vi "Parse Xeryon STAT.vi"(11 "STAT Word":i32) -> (2 "STAT True":string, 3 "STAT":string[][](table))   [LabVIEW 2019, in "Inst UI.Xeryon-Rotator.lvclass"]
uses:
  Inst UI.Xeryon-Rotator.lvclass
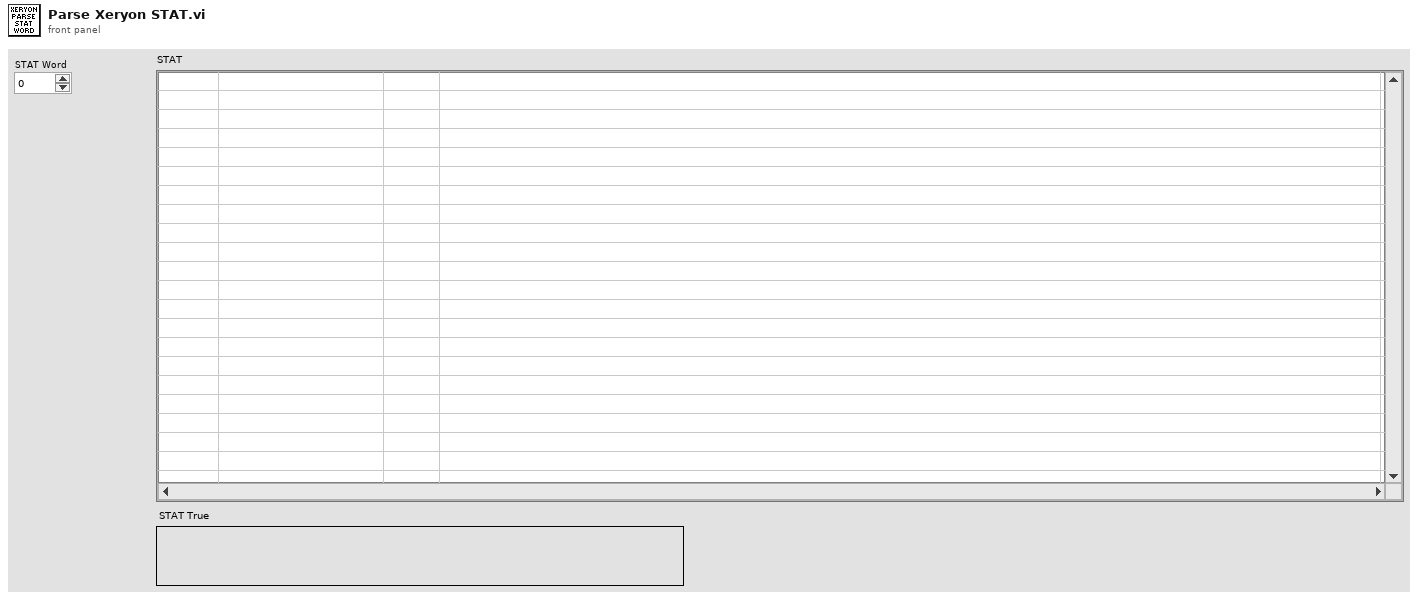
[diagram p1: front panel]
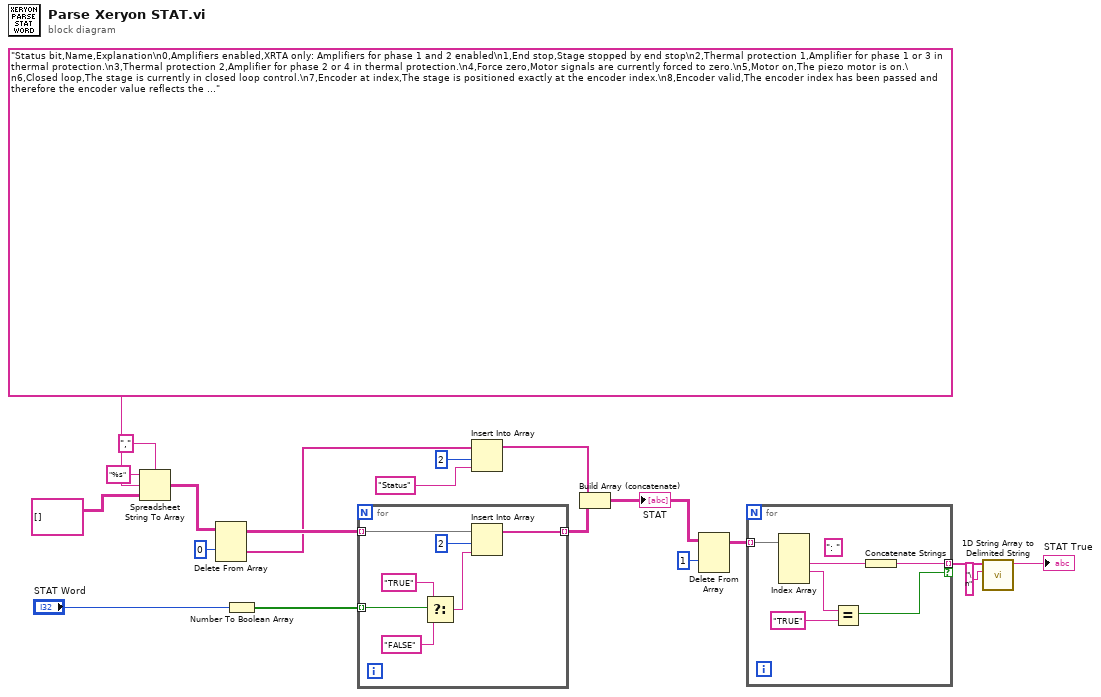
[diagram p0: block diagram]
diagram:
  n1 = Spreadsheet String To Array(delimiter (Tab)=",", format string="%s", spreadsheet string="Status bit,Name,Explanation\n0,Amplifiers enabled,XRTA only: Amplifiers for phase 1 and 2 enabled\n1,End stop,Stage stopped by end stop\n2,Thermal protection 1,Amplifier for phase 1 or 3 in thermal protection.\n3,Thermal protection 2,Amplifier for phase 2 or 4 in thermal protection.\n4,Force zero,Motor signals are currently forced to zero.\n5,Motor on,The piezo motor is on.\n6,Closed loop,The stage is currently in closed loop control.\n7,Encoder at index,The stage is positioned exactly at the encoder index.\n8,Encoder valid,The encoder index has been passed and therefore the encoder value reflects the absolute position and not the relative position with respect to the startup position.\n9,Searching index,The stage is currently searching the index position.\n10,Position reached,The target position is reached (within tolerance limits).\n11,Error compensation,Error compensation is on.\n12,Encoder error,There is an error produced by the encoder.\n13,Scanning,The stage is in a scanning mode.\n14,Left end stop,The left end stop is passed.\n15,Right end stop,The right end stop is passed.\n16,Error limit,The position error has reached the limit set by ELIM. This can indicate a collision or mechanical limit (end of stroke).\n17,Searching optimal frequency,The driver is searching for the optimal excitation frequency of the piezo motor.\n18,Safety timeout triggered,The safety timeout was triggered. See the explanation of the command 'TOU2'.\n19,EtherCAT acknowledge,Used when control via EtherCAT\n20,Emergency stop,not used\n21,Position fail,The safety timeout TOU3 was triggered.", array type (2D Dbl)=string[][] [] ("2-D Array")) -> (array=w5:string[][])
  n2 = Delete From Array(array=w5, index (row)=0) -> (deleted portion=w18:string[], array with subset deleted=w19:string[][])  [unwired: 2 in]
  n3 = Number To Boolean Array(number="STAT Word") -> (Boolean array=w2:bool[])
  n4 = for {
    tunnel: w19 -> [w24] mode=indexing
    tunnel: w2 -> [w27] mode=indexing
    tunnel: [w21] -> w14 mode=indexing
    n5 = Select(t="TRUE", s=w27, f="FALSE") -> (s? t:f=w23:string)
    n6 = Insert Into Array(array=w24, index=2, new element=w23) -> (w21:string[])
  }
  n7 = Insert Into Array(array=w18, index=2, new element="Status" ("new element/subarray")) -> (w15:string[])
  n8 = Build Array (concatenate)(w15, w14) -> (w1:string[][])
  "STAT" <- w1
  n9 = Delete From Array(array=w1, index (row)=1) -> (array with subset deleted=w12:string[][])  [unwired: 2 in, 1 out]
  n10 = for {
    tunnel: w12 -> [w33] mode=indexing
    tunnel: [w28] -> w11 mode=indexing if=w30
    (unwired) ": " ("string")
    n11 = Index Array(array=w33) -> (element #2=w29:string, element #3=w32:string)  [unwired: 4 in, 2 out]
    n12 = Equal?(x=w32, y="TRUE") -> (x = y?=w30:bool)
    n13 = Concatenate Strings(w29) -> (w28:string)
  }
  n14 = call <vilib>:"1D String Array to Delimited String.vi"("delimiter"="\n", "string array"=w11) -> ("delimited string"=→"STAT True":string)  [unwired: 9 in]
